vi "get entype settings.vi"(8 "error in (no error)":errorcluster, 10 "entype_settings":cluster{"EngineType":u32, "DriverType":u32}, 11 "id":i32) -> (0 "error out":errorcluster, 2 "entype_settings out":cluster{"EngineType":u32, "DriverType":u32}, 3 "function return":i32)   [LabVIEW 2012, in "libximc.lvlib"]
doc: "result_t XIMC_API get_entype_settings (device_t id, entype_settings_t* entype_settings);"
uses:
  libximc.lvlib
  libximc.dll
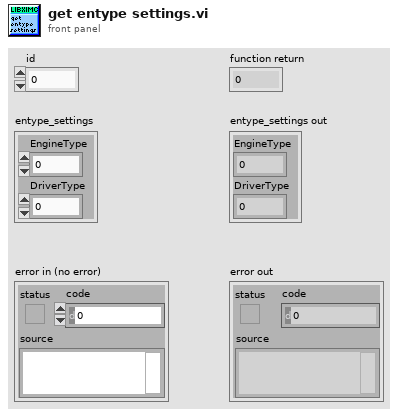
[diagram p1: front panel]
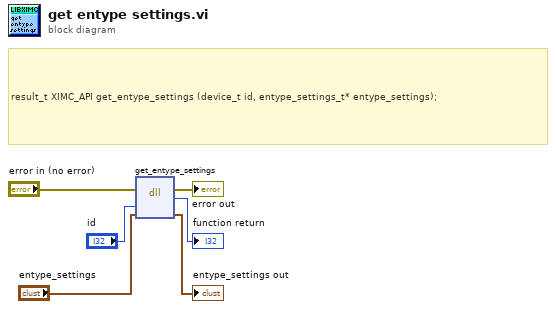
[diagram p0: block diagram]
diagram:
  # "result_t XIMC_API get_entype_settings (device_t id, entype_settings_t* entype_settings);"
  n1 = dll-call lib="C:/Users/Vasily/Att_examples/LabVIEW_example/libximc.*" fn="get_entype_settings"(error in="error in (no error)", "id"="id", "entype_settings"="entype_settings") -> (error out=→"error out":errorcluster, →"function return":i32, "entype_settings"=→"entype_settings out":cluster{"EngineType":u32, "DriverType":u32})  [unwired: 3 in, 1 out]
